vi "Write and read packed data to DRAM-host.vi"() -> ()   [LabVIEW 2015]
uses:
  <vilib>/rvi/interface/RandomDataEmulation/nirviRandomDataOpen.vi
  <vilib>/rvi/interface/common/niFpgaCacheSessionInfoDynamic.vi
  <vilib>/FPGAPlugInAG/Dynamic/niLvFpga_Reset_Dynamic.vi
  <vilib>/FPGAPlugInAG/Dynamic/niLvFpga_Run_Dynamic.vi
  <vilib>/Utility/error.llb/Error Cluster From Error Code.vi
  <vilib>/rvi/errors/niLvFpgaAdjustHostInterfaceError.vi
  <vilib>/FPGAPlugInAG/Dynamic/niLvFpga_Close_Dynamic.vi
  <vilib>/rvi/interface/nirviOpenFPGA/nirviOpenFPGA.xnode
  Other Test Codes/Write packed data to DRAM.vi
  <vilib>/rvi/interface/nirviMethod/nirviMethod.xnode
  <vilib>/rvi/interface/nirviReadWriteControl/nirviReadWriteControl.xnode
  <vilib>/rvi/interface/nirviCloseFPGA/nirviCloseFPGA.xnode
  <vilib>/rvi/errors/niLvFpgaMergeErrorWithErrorCode.vi
  <vilib>/FPGAPlugInAG/Dynamic/niLvFpga_ReadFifo_Dynamic.vi
  <vilib>/FPGAPlugInAG/Dynamic/niLvFpga_WriteFifo_Dynamic.vi
  NiFpgaLv.dll
  <vilib>/rvi/interface/Simulation/niFpgaSimulationCallBeginRW.vi
panel:
  out "Empty Elements Remaining":u32
  in  "Write DRAM enable?":bool
  out "read DRAM done?":bool
  out "Write DRAM done?":bool
  out "Data readed":u32
  out "Data":u32[](array[numeric])
  in  "Total elements to write":i32
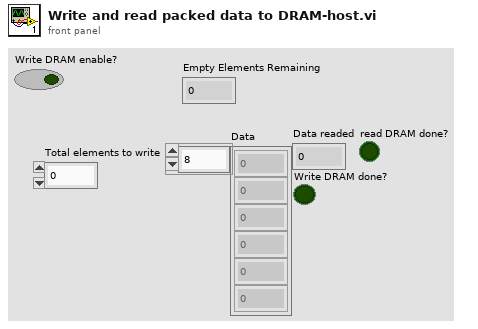
[diagram p1: front panel]
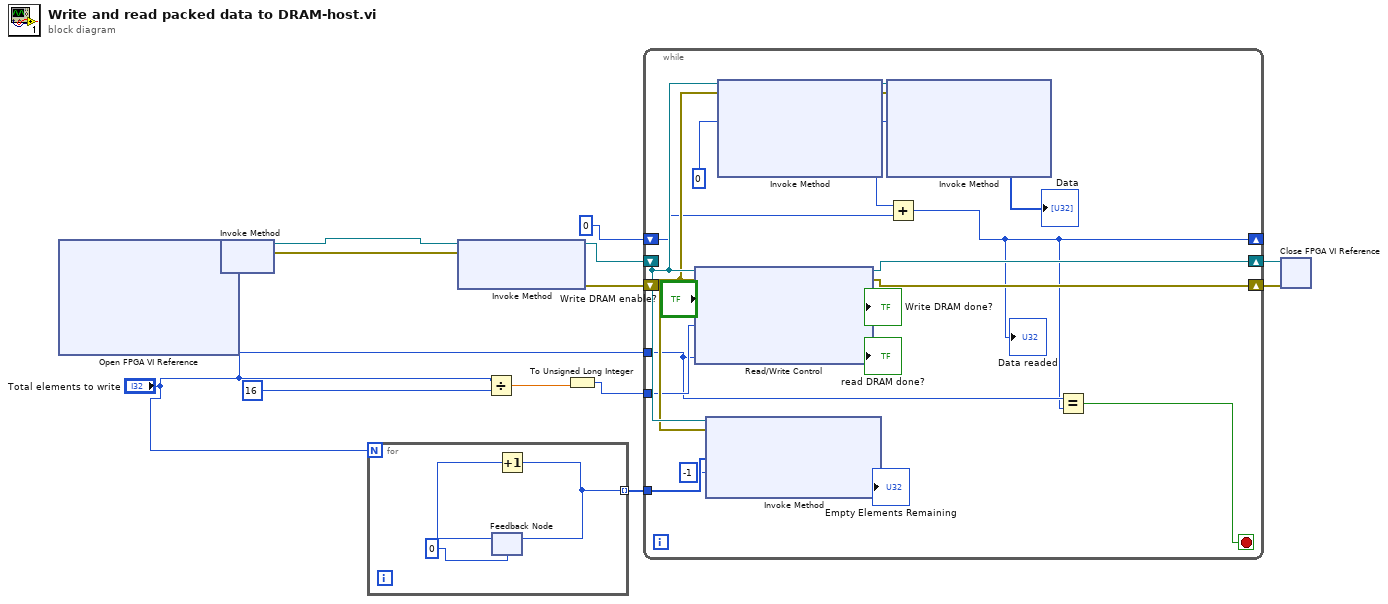
[diagram p0: block diagram]
diagram:
  n1 = xnode "Open FPGA VI Reference"() -> ("FPGA VI引用输出"=w14:refnum<k20>, "错误输出"=w13:errorcluster)  [unwired: 2 in]
  n2 = xnode "Invoke Method"("FPGA VI引用输入"=w14, "错误输入"=w13) -> ("FPGA VI引用输出"=w2:refnum<k20>, "错误输出"=w1:errorcluster)
  n3 = for {
    N: "Total elements to write" -> [_]
    tunnel: [w15] -> w8 mode=indexing
    n4 = feedback #1(u32 0) -> (w17:u32)
    n5 = Increment(x=w17) -> (x+1=w15:u32)
    n6 = feedback-in #1(w15) -> ()
  }
  n7 = xnode "Invoke Method"("FPGA VI引用输入"=w2, "错误输入"=w1) -> ("FPGA VI引用输出"=w10:refnum<k20>, "错误输出"=w9:errorcluster)  [unwired: 1 in]
  n8 = Divide(x="Total elements to write", y=16) -> (x/y=w6:dbl)
  n9 = To Unsigned Long Integer(number=w6) -> (unsigned 32bit integer=w3:u32)
  n10 = while {
    tunnel: "Total elements to write" -> [w24]
    tunnel: w8 -> [w34]
    shift-right: [w37] -> w12
    shift-left: w10 -> [w32]
    shift-right: [w36] -> w11
    shift-left: w9 -> [w31]
    tunnel: w3 -> [w26]
    shift-right: [w19] -> _
    shift-left: u32 0 -> [w20]
    stop <- w23 stop-if-true
    n11 = xnode "Read/Write Control"("FPGA VI引用输入"=w32, "错误输入"=w31, "Write DRAM enable?"="Write DRAM enable?", "Total packed data to write?"=w26, "Total elements to write"=w24) -> ("FPGA VI引用输出"=w37:refnum<k20>, "错误输出"=w36:errorcluster, "Write DRAM done?"=→"Write DRAM done?":bool, "read DRAM done?"=→"read DRAM done?":bool)
    n12 = xnode "Invoke Method"("FPGA VI引用输入"=w32, "错误输入"=w31, "Data"=w34, "Timeout (ms)"=-1) -> ("Empty Elements Remaining"=→"Empty Elements Remaining":u32)  [unwired: 2 out]
    n13 = xnode "Invoke Method"("FPGA VI引用输入"=w32, "错误输入"=w31, "Number of Elements"=u32 0) -> ("FPGA VI引用输出"=w29:refnum<k20>, "错误输出"=w28:errorcluster, "Elements Remaining"=w25:u32)  [unwired: 1 in, 1 out]
    n14 = xnode "Invoke Method"("FPGA VI引用输入"=w29, "错误输入"=w28, "Number of Elements"=w25) -> ("Data"=→"Data":u32[])  [unwired: 1 in, 3 out]
    n15 = Add(x=w25, y=w20) -> (x+y=w19:u32)
    "Data readed" <- w19
    n16 = Equal?(x=w24, y=w19) -> (x = y?=w23:bool)
  }
  n17 = xnode "Close FPGA VI Reference"("FPGA VI Reference In"=w12, "error in"=w11) -> ()  [unwired: 1 out]
